vi "HookValidationA1.vi"(9 "中心到镜像产品连线角度":dbl format="%#_3g", 11 "各槽角":dbl[](array[numeric])) -> (0 "槽角序号":i32, 1 "槽在中心到产品连线所在侧":enum16{"左侧-逆时针向", "右侧-顺时针向"}(ring), 3 "指向最接近的中心位槽角":dbl format="%#_3g")   [LabVIEW 2018]
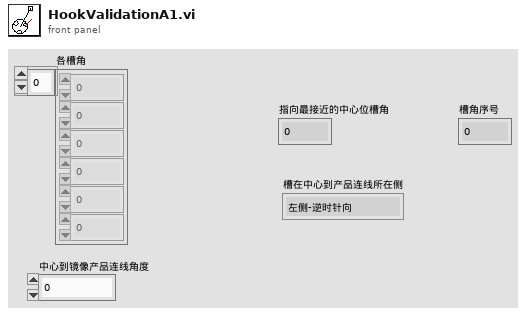
[diagram p1: front panel]
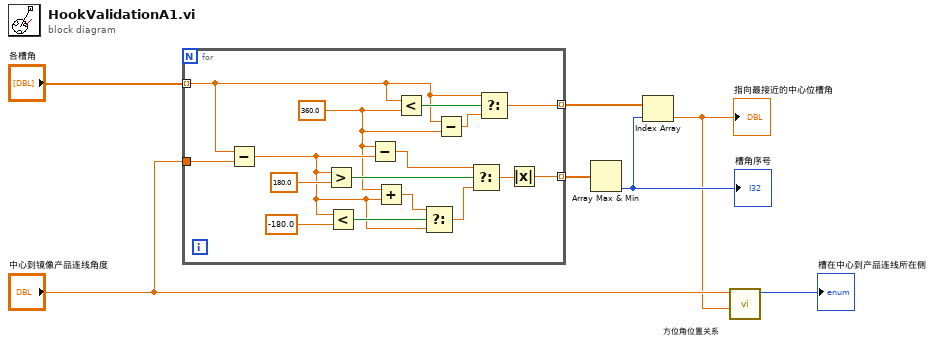
[diagram p0: block diagram]
diagram:
  n1 = for {
    tunnel: "中心到镜像产品连线角度" -> [w23]
    tunnel: [w13] -> w7 mode=indexing
    tunnel: [w9] -> w6 mode=indexing
    tunnel: "各槽角" -> [w8] mode=indexing
    w11 = 360.0 ("x")
    n2 = Subtract(x=w8, y=w23) -> (x-y=w15:dbl)
    n3 = Greater?(x=w15, y=180.0) -> (0:w21:bool)
    n4 = Less?(x=w15, y=-180.0) -> (x < y?=w17:bool)
    n5 = Subtract(x=w11, y=w15) -> (x-y=w20:dbl)
    n6 = Add(x=w11, y=w15) -> (x+y=w18:dbl)
    n7 = Less?(x=w8, y=w11) -> (x < y?=w12:bool)
    n8 = Select(t=w18, s=w17, f=w15) -> (s? t:f=w16:dbl)
    n9 = Subtract(x=w8, y=w11) -> (x-y=w10:dbl)
    n10 = Select(t=w20, s=w21, f=w16) -> (s? t:f=w14:dbl)
    n11 = Select(t=w8, s=w12, f=w10) -> (s? t:f=w9:dbl)
    n12 = Absolute Value(x=w14) -> (abs(x)=w13:dbl)
  }
  n13 = Array Max & Min(array=w7) -> (min index (indices)=w5:i32)  [unwired: 3 out]
  "槽角序号" <- w5
  n14 = Index Array(array=w6, index=w5) -> (element=w1:dbl)
  "指向最接近的中心位槽角" <- w1
  n15 = call "方位角位置关系.vi"("输入角度"=w1, "基准角度"="中心到镜像产品连线角度") -> ("输入角相对基准角的方位"=→"槽在中心到产品连线所在侧":enum16{"左侧-逆时针向", "右侧-顺时针向"})  [unwired: 9 in]
